vi "Retrieve Taus.vi"(8 "error in":errorcluster, 10 "Ringdowns":i16[][](array[numeric]), 11 "CRDS Cell in":refnum<class "CRDS Cell.lvclass">) -> (0 "error out":errorcluster, 2 "Request Restart?":bool, 3 "CRDS Cell out":refnum<class "CRDS Cell.lvclass">)   [LabVIEW 2015, in "CRDS Cell.lvclass"]
doc: "Takes the ringdown data for the cell acquired over a 1 s period and retrieves the averaged tau based on the average of the shot fits. This VI will also populate the statistics in the extinction cluster and provide both a decimated trace and a decimated trace for the fit using the A, B and tau parameters retrieved.\n\nAll math is linear - no errors are thrown except potentially in accessors for CRDS data."
uses:
  CRDS Cell.lvclass
  CRDS Cell.lvclass/CRDS Cell.ctl
  Data/Cell/CRDS Cell Data.lvclass/CRDS Cell Data.ctl
  <vilib>/Analysis/baseanly.llb/Mean (DBL).vi
  Data/Cell/Read extParam.vi
  Data/Cell/Write extParam.vi
  Data/Cell/Write Ringdowns.vi
  Data/Cell/CRDS Cell Data.lvclass
  <vilib>/Analysis/NI_AALBase.lvlib
  General/Math Utilities.lvlib
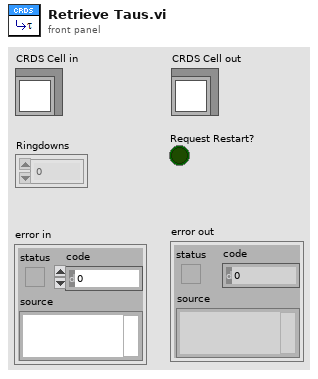
[diagram p1: front panel]
types:
  T1 = typedef "extparam.ctl" = cluster{"Tau":sgl, "Tau0cor":sgl, "ext":sgl, "extCorr":sgl, "stdevTau":sgl, "eTau":sgl, "taucorr":sgl, "Tau0":sgl, "max":sgl}
  T2 = typedef "Get Tau Method.ctl" = enum8{"DFT-1", "DFT-5", "LRS"}
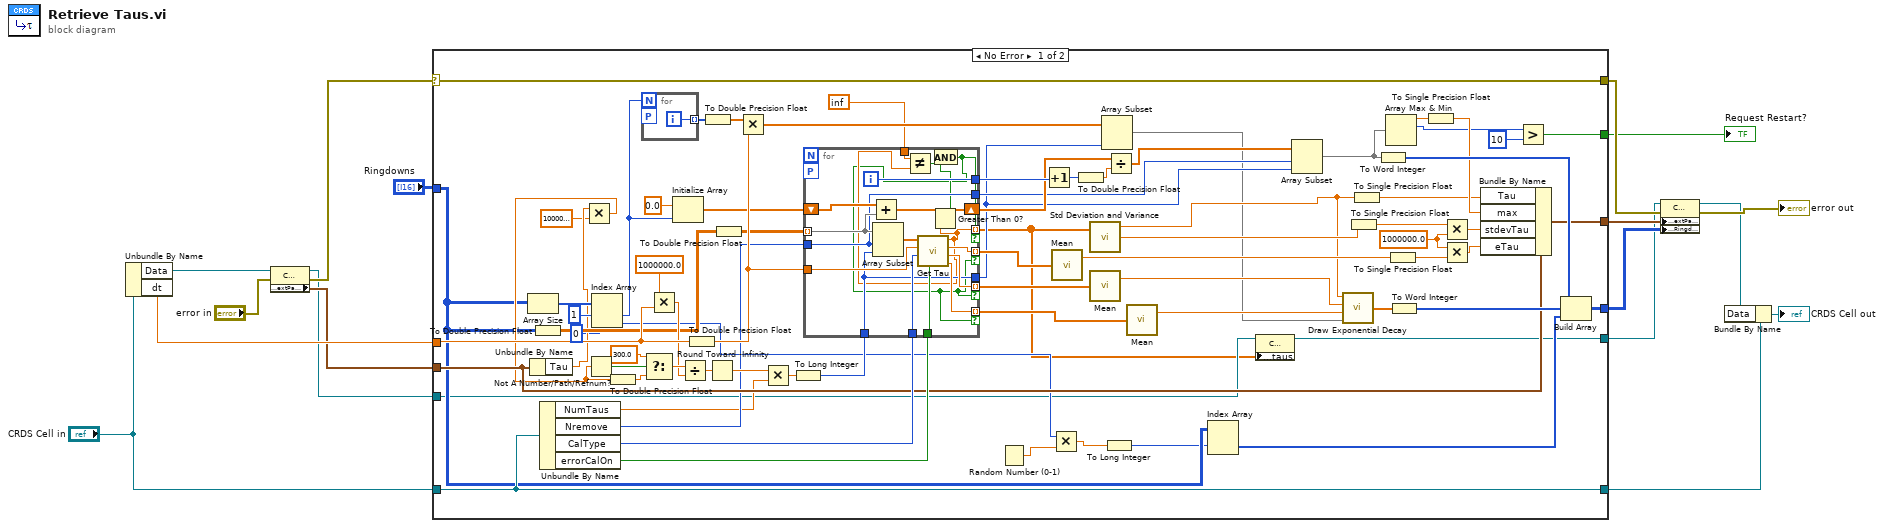
[diagram p0: block diagram]
diagram:
  n1 = Unbundle By Name("CRDS Cell in") -> ("Data"=w11:refnum<class "CRDS Cell Data.lvclass">, "dt"=w7:dbl)
  n2 = property class="CRDS Cell"(reference=w11, error in="error in") -> (reference out=w2:refnum<class "CRDS Cell Data.lvclass">, error out=w13:errorcluster, "Data Access:extParam"=w4:T1)
  n3 = case shown="No Error" w13 {
    selector: w13 -> [w41 w115]
    tunnel: [w41 w115] -> w16
    tunnel: [w40 w114] -> w9
    tunnel: "CRDS Cell in" -> [w40 w114]
    tunnel: "Ringdowns" -> [w23 _]
    tunnel: w7 -> [w49 _]
    tunnel: w4 -> [w60 _]
    tunnel: [w61 _] -> w6
    tunnel: [w56 _] -> w17
    tunnel: [w33 _] -> w3
    tunnel: w2 -> [w20 w113]
    tunnel: [w18 w113] -> w1
    frame No Error {
      w44 = sgl 1000000.0
      n4 = Array Size(array=w23) -> (size(s)=w78:i32[])
      n5 = Unbundle By Name(w60) -> ("Tau"=w31:sgl)
      n6 = To Double Precision Float(number=w23) -> (double precision float=w38:dbl[][])
      n7 = Unbundle By Name(w40) -> ("NumTaus"=w35:sgl, "Nremove"=w36:i32, "CalType"=w63:T2, "errorCalOn"=w62:bool)
      n8 = Multiply(x=w31, y=sgl 1000000.0) -> (x*y=w29:sgl)
      n9 = Not A Number/Path/Refnum?(number/path/refnum=w29) -> (NaN/Path/Refnum?=w68:bool)
      n10 = Index Array(array=w78, index #1=1 ("index"), index #2=0 ("index")) -> (element #1=w64:i32, element #2=w25:i32)
      n11 = To Double Precision Float(number=w29) -> (double precision float=w39:dbl)
      n12 = for {
        N: w64 -> [_]
        tunnel: [w112] -> w82 mode=indexing
        workers-P: _ -> [_]
        i -> [w112]
      }
      n13 = Select(t=300.0, s=w68, f=w39) -> (s? t:f=w66:dbl)
      n14 = Multiply(x=1000000.0, y=w49) -> (x*y=w47:dbl)
      n15 = Initialize Array(0.0 ("element"), w64) -> (w73:dbl[])
      n16 = Divide(x=w66, y=w47) -> (x/y=w77:dbl)
      n17 = To Double Precision Float(number=w49) -> (double precision float=w92:dbl)
      n18 = To Double Precision Float(number=w82) -> (double precision float=w81:dbl[])
      n19 = Round Toward -Infinity(1:w77) -> (0:w85:dbl)
      n20 = To Double Precision Float(number=w38) -> (double precision float=w37:dbl[][])
      n21 = Multiply(x=w81, y=w92) -> (x*y=w52:dbl[])
      n22 = Multiply(x=w85, y=w35) -> (x*y=w89:dbl)
      n23 = To Long Integer(number=w89) -> (32bit integer=w65:i32)
      n24 = for {
        tunnel: [w97] -> w19 mode=indexing if=w94
        tunnel: w37 -> [w105] mode=indexing
        tunnel: [w111] -> w69 mode=indexing if=w94
        tunnel: [w110] -> w70 mode=indexing if=w94
        tunnel: [w109] -> w71 mode=indexing if=w94
        shift-right: [w108] -> w74
        shift-left: w73 -> [w106]
        tunnel: w92 -> [w107]
        tunnel: [w99] -> w80
        tunnel: w65 -> [w101]
        workers-P: _ -> [_]
        tunnel: w63 -> [w103]
        tunnel: w62 -> [w102]
        tunnel: [w100] -> w53
        tunnel: [w101] -> w51
        tunnel: w36 -> [w100]
        tunnel: inf -> [w96]
        i -> [w99]
        n25 = Add(x=w106, y=w105) -> (x+y=w108:dbl[])
        n26 = Array Subset(array=w105, index=w100, length=w101) -> (w104:dbl[])
        n27 = call "Get Tau.vi"("ErrorCallOn"=w102, "CalType"=w103, "Dt"=w107, "X"=w104) -> ("B"=w109:dbl, "A"=w110:dbl, "e_tau"=w111:dbl, "tau"=w97:dbl)  [unwired: 4 in]
        n28 = Not Equal?(x=w96, y=w97) -> (x != y?=w95:bool)
        n29 = Greater Than 0?(x=w97) -> (x > 0?=w98:bool)
        n30 = And(x=w95, y=w98) -> (x .and. y?=w94:bool)
      }
      n31 = Random Number (0-1)() -> (number: 0 to 1=w26:dbl)
      n32 = Increment(x=w80) -> (x+1=w87:i32)
      n33 = Multiply(x=w25, y=w26) -> (x*y=w24:dbl)
      n34 = call-poly <vilib>:"Mean.vi"("X"=w69) -> ("mean"=w83:dbl)  [unwired: 1 out]
      n35 = To Double Precision Float(number=w87) -> (double precision float=w86:dbl)
      n36 = call <vilib>:"Std Deviation and Variance.vi"("X"=w19) -> ("mean"=w55:dbl, "standard deviation"=w84:dbl)  [unwired: 1 in, 1 out]
      n37 = call-poly <vilib>:"Mean.vi"("X"=w70) -> ("mean"=w75:dbl)  [unwired: 1 out]
      n38 = Array Subset(array=w52, length=w51) -> (w50:dbl[])  [unwired: 1 in]
      n39 = To Long Integer(number=w24) -> (32bit integer=w22:i32)
      n40 = Divide ("mean")(x=w74, y=w86) -> (x/y=w54:dbl[])
      n41 = call-poly <vilib>:"Mean.vi"("X"=w71) -> ("mean"=w76:dbl)  [unwired: 1 out]
      n42 = Index Array(array=w23, index (row)=w22) -> (element=w21:i16[])  [unwired: 1 in]
      n43 = property class="CRDS Cell"(reference=w20, "Data Access:taus"=w19) -> (reference out=w18:refnum<class "CRDS Cell Data.lvclass">)  [unwired: 1 in, 1 out]
      n44 = Array Subset(array=w54, index=w53, length=w51) -> (w42:dbl[])
      n45 = call "Draw Exponential Decay.vi"("time"=w50, "B"=w76, "A"=w75, "tau"=w55) -> ("ExponentialOut"=w46:dbl[])
      n46 = To Single Precision Float(number=w84) -> (single precision float=w45:sgl)
      n47 = To Single Precision Float(number=w55) -> (single precision float=w43:sgl)
      n48 = To Word Integer(number=w42) -> (16bit integer=w90:i16[])
      n49 = Array Max & Min(array=w42) -> (max value=w93:dbl, max index (indices)=w32:i32)  [unwired: 2 out]
      n50 = To Single Precision Float(number=w83) -> (single precision float=w88:sgl)
      n51 = To Word Integer(number=w46) -> (16bit integer=w91:i16[])
      n52 = To Single Precision Float(number=w93) -> (single precision float=w59:sgl)
      n53 = Multiply(x=w45, y=w44) -> (x*y=w58:sgl)
      n54 = Multiply(x=w44, y=w88) -> (x*y=w57:sgl)
      n55 = Bundle By Name(cluster=w60, "Tau"=w43, "max"=w59, "stdevTau"=w58, "eTau"=w57) -> (w56:T1)
      n56 = Greater?(x=w32, y=10) -> (0:w33:bool)
      n57 = Build Array(w90, w91, w21) -> (w61:i16[][])
    }
    frame Error {
    }
  }
  "Request Restart?" <- w3
  n58 = property class="CRDS Cell"(reference=w1, error in=w16, "Data Access:extParam"=w17, "Data Access:Ringdowns"=w6) -> (reference out=w10:refnum<class "CRDS Cell Data.lvclass">, error out=→"error out":errorcluster)
  n59 = Bundle By Name(cluster=w9, "Data"=w10) -> (→"CRDS Cell out":refnum<class "CRDS Cell.lvclass">)
